vi "BRig_dataTrial_T_ENL2.vi"() -> (2 "output_T_ENL2":i32)   [LabVIEW 2014]
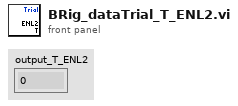
[diagram p1: front panel]
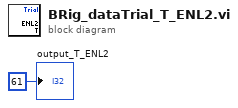
[diagram p0: block diagram]
diagram:
  "output_T_ENL2" <- 61 ("output_iBlock")
